vi "check user test.vi"() -> ()   [LabVIEW 2020]
uses:
  <vilib>/Spiers New Technologies/SNT/Alfred-Connector/Utilities/Login Data Input.ctl
  <vilib>/Spiers New Technologies/SNT/Alfred-Connector/Utilities/Login Info Return.ctl
  <vilib>/Spiers New Technologies/SNT/Alfred-Connector/Alfred.lvlib
panel:
  in  "stop":bool
  out "User ID":string
  out "Login Info":T1
  out "Valid?":bool
  in  "Login Method":enum16{"User ID/PW", "Badge"}(ring)
  in  "Login Data Input":T2={"Username"="", "Badge"="3B 88 01 00 03 08 06 66 00 77 80 78", "Password"="", "Privilege"="Test Stand Capstone Leak Test"}
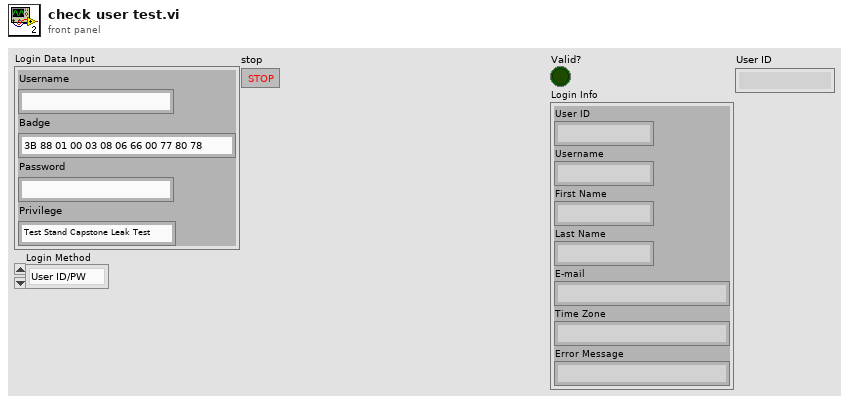
[diagram p1: front panel]
types:
  T1 = typedef "Alfred.lvlib/Login Info Return.ctl" = cluster{"User ID":string, "Username":string, "First Name":string, "Last Name":string, "E-mail":string, "Time Zone":string, "Error Message":string}
  T2 = typedef "Alfred.lvlib/Login Data Input.ctl" = cluster{"Username":string, "Badge":string, "Password":string, "Privilege":string}
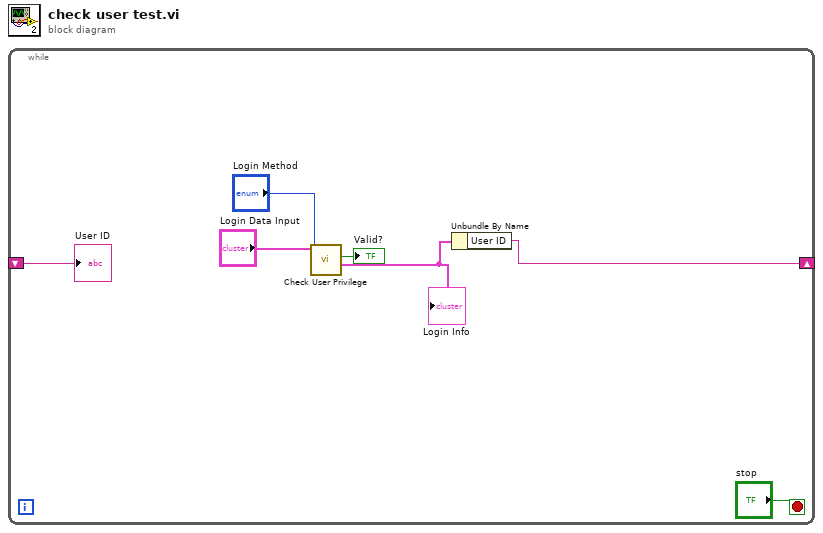
[diagram p0: block diagram]
diagram:
  n1 = while {
    shift-right: [w3] -> _
    shift-left: _ -> [w2]
    stop <- "stop" stop-if-true
    n2 = call <vilib>:"Check User Privilege.vi"("Login Method"="Login Method", "Login Data Input"="Login Data Input") -> ("Login Info"=w4:T1, "Valid?"=→"Valid?":bool)  [unwired: 7 in, 1 out]
    "Login Info" <- w4
    n3 = Unbundle By Name(w4) -> ("User ID"=w3:string)
    "User ID" <- w2
  }
